vi "CTRE_PigeonIMU_SetTempCompensationEnable.vi"(8 "error in (no error)":errorcluster, 10 "Enable?":bool=TRUE, 11 "PigeonIMUDevRef":T1={"DeviceStatus"={"status"=FALSE, "code"=0, "source"=""}, "Device Number"=0, "Type"=352321536, "Device ID"=0, "Handle"=0, "UsageFrame"=0, "Library Path"=path ""} {"Type" items=["CAN"=352321536, "TalonSRX"=33554432]}) -> (0 "error out":errorcluster, 3 "PigeonIMUDevRef Out":T1={"DeviceStatus"={"status"=FALSE, "code"=0, "source"=""}, "Device Number"=0, "Type"=352321536, "Device ID"=0, "Handle"=0, "UsageFrame"=0, "Library Path"=path ""} {"Type" items=["CAN"=352321536, "TalonSRX"=33554432]})   [LabVIEW 2016]
uses:
  CTRE_PigeonIMU_DeviceRef.ctl
  CTRE_PigeonIMU_ConnectionType.ctl
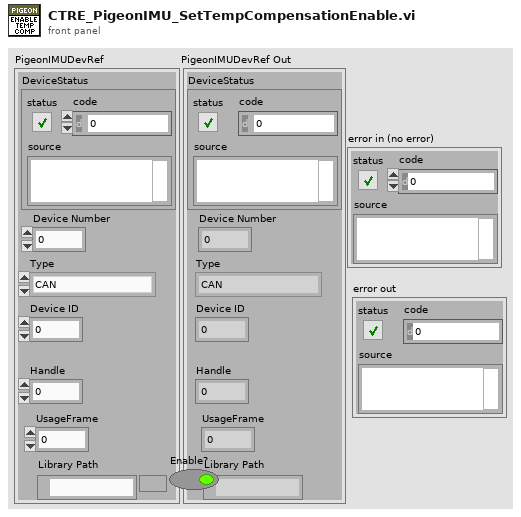
[diagram p1: front panel]
types:
  T1 = typedef "CTRE_PigeonIMU_DeviceRef.ctl" = cluster{"DeviceStatus":errorcluster, "Device Number":u8, "Type":T2, "Device ID":u32, "Handle":u64, "UsageFrame":u32, "Library Path":path}
  T2 = typedef "CTRE_PigeonIMU_ConnectionType.ctl" = u32
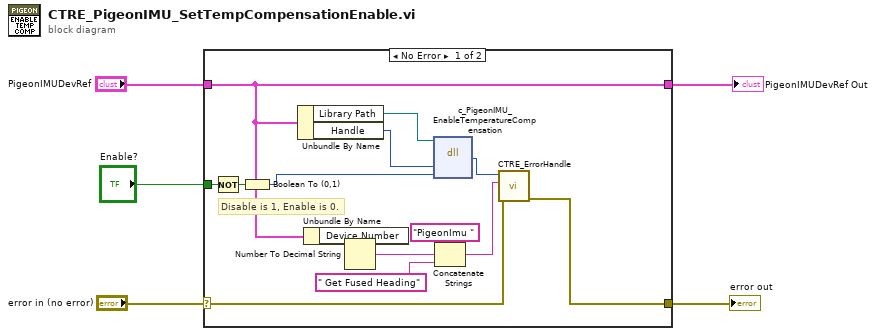
[diagram p0: block diagram]
diagram:
  n1 = case shown="No Error" "error in (no error)" {
    selector: "error in (no error)" -> [w7 w20]
    tunnel: [w6 w20] -> w4
    tunnel: [w9 w21] -> w2
    tunnel: "PigeonIMUDevRef" -> [w9 w21]
    tunnel: "Enable?" -> [w19 _]
    frame No Error {
      # "Disable is 1, Enable is 0."
      n2 = Not(x=w19) -> (.not. x?=w18:bool)
      n3 = Boolean To (0,1)(Boolean=w18) -> (0, 1=w15:i16)
      n4 = Unbundle By Name(w9) -> ("Library Path"=w17:path, "Handle"=w16:u64)
      n5 = Unbundle By Name(w9) -> ("Device Number"=w13:u8)
      n6 = Number To Decimal String(number=w13) -> (decimal integer string=w12:string)  [unwired: 1 in]
      n7 = dll-call lib="?" fn="c_PigeonIMU_EnableTemperatureCompensation"(path in=w17, "handle"=w16, "bTempCompEnable"=w15) -> ("return type"=w14:i32)  [unwired: 4 in, 2 out]
      n8 = Concatenate Strings("PigeonImu " ("string"), w12, " Get Fused Heading" ("string")) -> (w8:string)
      n9 = call "CTRE_ErrorHandle.vi"("error in"=w7, "origin"=w8, "code"=w14) -> ("error out"=w6:errorcluster)  [unwired: 8 in]
    }
    frame Error {
    }
  }
  "PigeonIMUDevRef Out" <- w2
  "error out" <- w4
